vi "Trim Whitespace.vi"(0 "string":string caption="String", 1 "location (both)":T1 caption="Position (beide)" items=["beide", "Stringanfang", "Stringende"]) -> (2 "trimmed string":string caption="gekürzter String")   [LabVIEW 2009]
doc: "Entfernt sämtliche leeren Zwischenräume (Leerstellen, Tabs, Zeilenumbrüche und Zeilenvorschübe) vom Anfang, vom Ende oder von beiden Enden des <B>Strings</B>."
uses:
  whitespace.ctl
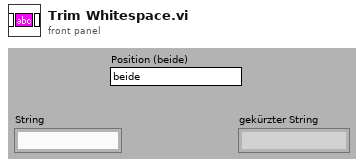
[diagram p1: front panel]
types:
  T1 = typedef "whitespace.ctl" = u16
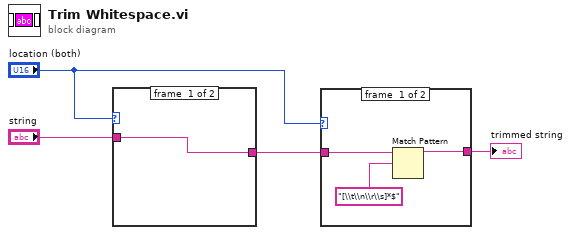
[diagram p0: block diagram]
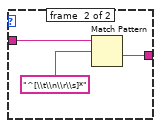
[diagram p3: hidden frame]
diagram:
  n1 = case shown="0, 1" "location (both)" {
    tunnel: [w5 w8] -> w3
    tunnel: "string" -> [w5 w6]
    frame #0 {
    }
    frame #1 {
      n2 = Match Pattern(string=w6, regular expression="^[\\t\\n\\r\\s]*") -> (after substring=w8:string)  [unwired: 1 in, 3 out]
    }
  }
  n3 = case shown="0, 2" "location (both)" {
    tunnel: [w11 w12] -> w4
    tunnel: w3 -> [w10 w12]
    frame #0 {
      n4 = Match Pattern(string=w10, regular expression="[\\t\\n\\r\\s]*$") -> (before substring=w11:string)  [unwired: 1 in, 3 out]
    }
    frame #1 {
    }
  }
  "trimmed string" <- w4
